vi "Get Group Mappings.vi"(8 "error in":errorcluster, 11 "session reservation in":refnum<class "Session Reservation.lvclass">) -> (0 "error out":errorcluster, 1 "group mappings":T1, 3 "session reservation out":refnum<class "Session Reservation.lvclass">)   [LabVIEW 2020, in "Plug-In SDK Session Management V1.lvlib" / "Session Reservation.lvclass"]
doc: "Gets the group mappings for the session reservation."
uses:
  Session Reservation.lvclass
  Group Mapping.ctl
  Session Reservation.lvclass/Session Reservation.ctl
  Measurements/Helpers/Error Strings Global Internal.vi
  <vilib>/Utility/error.llb/Error Cluster From Error Code.vi
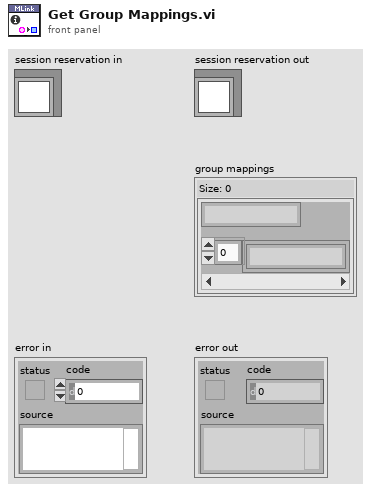
[diagram p1: front panel]
types:
  T1 = typedef "Plug-In SDK Session Management V1.lvlib/Session Reservation.lvclass/Group Mapping.ctl" = map{string, string[]}
  T2 = typedef "Plug-In SDK Session Management V1.lvlib/Session Reservation.lvclass/Data.ctl" = cluster{"session and driver infos":T3[], "pin or relay names":string[], "connection map":refnum<class "Connection Map.lvclass">, "pin map context":T8, "reservation observer":refnum<class "IReservation Observer.lvclass">, "dvr valid":bool, "group mappings":T1}
  T3 = typedef "Plug-In SDK Session Management V1.lvlib/Session Reservation.lvclass/Session and Driver Info.ctl" = cluster{"session info":T4, "session":variant, "session factory":refnum<class "ISession Factory.lvclass">, "initialize and close session behavior":T7}
  T4 = typedef "ni.measurementlink.sessionmanagement.v1.lvlib/ni_measurementlink_sessionmanagement_v1_SessionInformation.ctl" = cluster{"session":T5, "resource_name":string, "channel_list":string, "instrument_type_id":string, "session_exists":bool, "channel_mappings":T6[]}
  T5 = typedef "ni.measurementlink.sessionmanagement.v1.lvlib/nidevice_grpc_Session.ctl" = cluster{"name":string}
  T6 = typedef "ni.measurementlink.sessionmanagement.v1.lvlib/ni_measurementlink_sessionmanagement_v1_ChannelMapping.ctl" = cluster{"pin_or_relay_name":string, "site":i32, "channel":string, "multiplexer_resource_name":string, "multiplexer_route":string}
  T7 = typedef "Instrument Sessions.lvlib/ISession Factory.lvclass/Initialize and Close Session Behavior.ctl" = enum16{"Initialize and Close", "Attach and Detach", "Initialize and Detach", "Attach and Close"}
  T8 = typedef "ni.measurementlink.sessionmanagement.v1.lvlib/ni_measurementlink_PinMapContext.ctl" = cluster{"pin_map_id":string, "sites":i32[]}
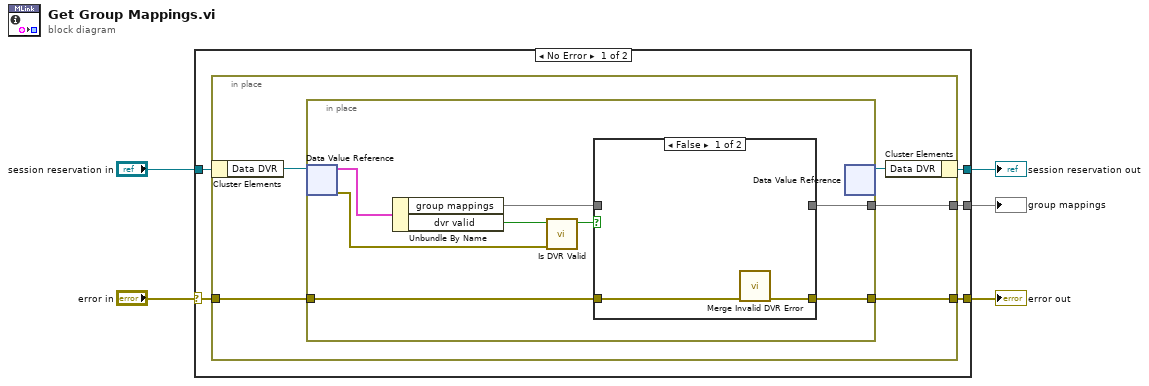
[diagram p0: block diagram]
diagram:
  n1 = case shown="No Error" "error in" {
    selector: "error in" -> [w7 w29]
    tunnel: "session reservation in" -> [w10 w28]
    tunnel: [w9 w28] -> w4
    tunnel: [w8 w29] -> w3
    tunnel: [w6 _] -> w1
    frame No Error {
      n2 = in-place {
        in-place-border: [w15] -> w8
        in-place-border: w7 -> [w12]
        in-place-border: [w11] -> w6
        n3 = in-place-cluster #1(w10) -> ("Data DVR"=w14:refnum<data-value>)
        n4 = in-place {
          in-place-border: w12 -> [w23]
          in-place-border: [w22] -> w15
          in-place-border: [w16] -> w11
          n5 = in-place-dvr #2(w14) -> (w20:T2, w17:errorcluster)
          n6 = Unbundle By Name(w20) -> ("group mappings"=w21:T1, "dvr valid"=w19:bool)
          n7 = call "Is DVR Valid.vi"("dvr error in"=w17, "dvr valid in"=w19) -> ("dvr valid out"=w18:bool)  [unwired: 9 in]
          n8 = case shown="False" w18 {
            tunnel: w23 -> [w25 w27]
            tunnel: [w24 w27] -> w22
            tunnel: w21 -> [_ w26]
            tunnel: [_ w26] -> w16
            frame False {
              n9 = call "Merge Invalid DVR Error.vi"("error in"=w25) -> ("error out"=w24:errorcluster)  [unwired: 10 in]
            }
            frame True {
            }
          }
          n10 = in-place-dvr #2() -> (w13:refnum<data-value>)  [unwired: 1 in, 1 out]
        }
        n11 = in-place-cluster #1("Data DVR"=w13) -> (w9:refnum<class "Session Reservation.lvclass">)
      }
    }
    frame Error {
    }
  }
  "error out" <- w3
  "session reservation out" <- w4
  "group mappings" <- w1
